vi "helper-collect-wind-direction.vi"(8 "error in":errorcluster, 10 "Result Virtual Name":string, 11 "Value in":dbl) -> (0 "error out":errorcluster, 1 "BUF Node":T1={"ADDR"=0, "Label"="", "Type"=enum."DI", "Mode"=enum."RIO", "Value"="", "Tags"="", "calibration"=[]} {"calibration"."Y" format="%#.3f"; "calibration"."X" format="%#.3f"; "ADDR" format="%04d"}, 2 "Result Node":T1={"ADDR"=0, "Label"="", "Type"=enum."DI", "Mode"=enum."RIO", "Value"="", "Tags"="", "calibration"=[]} {"calibration"."Y" format="%#.3f"; "calibration"."X" format="%#.3f"; "ADDR" format="%04d"}, 3 "Result":dbl)   [LabVIEW 2024]
uses:
  controls/IONode.ctl
  controls/type.address.ctl
  controls/enum.io.type.ctl
  controls/enum.io.mode.ctl
  controls/typeXyPoint.ctl
  controls/enumVarCtrlIO.ctl
  <vilib>/Utility/error.llb/Trim Whitespace.vi
  <vilib>/Utility/error.llb/Trim Whitespace One-Sided.vi
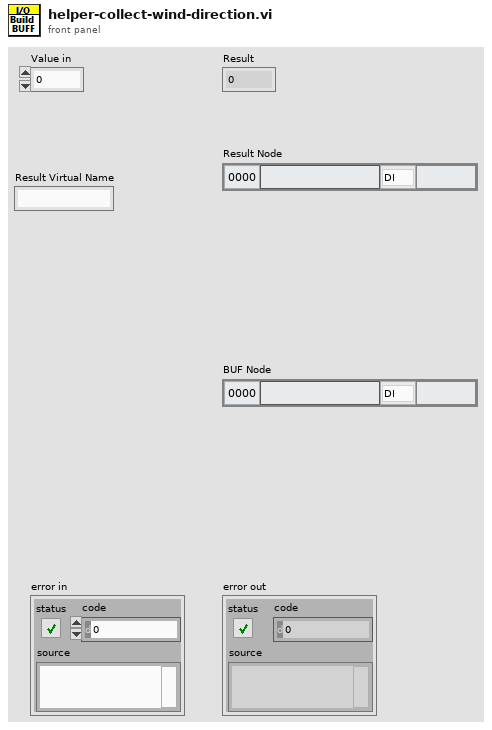
[diagram p1: front panel]
types:
  T1 = typedef "IONode.ctl" = cluster{"ADDR":T2, "Label":string, "Type":T3, "Mode":T4, "Value":string, "Tags":string, "calibration":T5[]}
  T2 = typedef "type.address.ctl" = u16
  T3 = typedef "enum.io.type.ctl" = enum16{"Type", "DI", "DO", "AI", "AO", "VL", "BUF"}
  T4 = typedef "enum.io.mode.ctl" = enum16{"Mode", "RIO", "SIM"}
  T5 = typedef "typeXyPoint.ctl" = cluster{"X":dbl, "Y":dbl}
  T6 = typedef "enumVarCtrlIO.ctl" = enum16{"IO Get By Key", "IO List Configs", "IO Add By Key", "IO Modify Value By Key", "IO Modify Calib By Key", "IO Modify ADDR By Key", "IO Modify Mode By Key", "IO Modify Type By Key", "IO Modify Name By Key", "IO Remove By Key", "IO Remove All"}
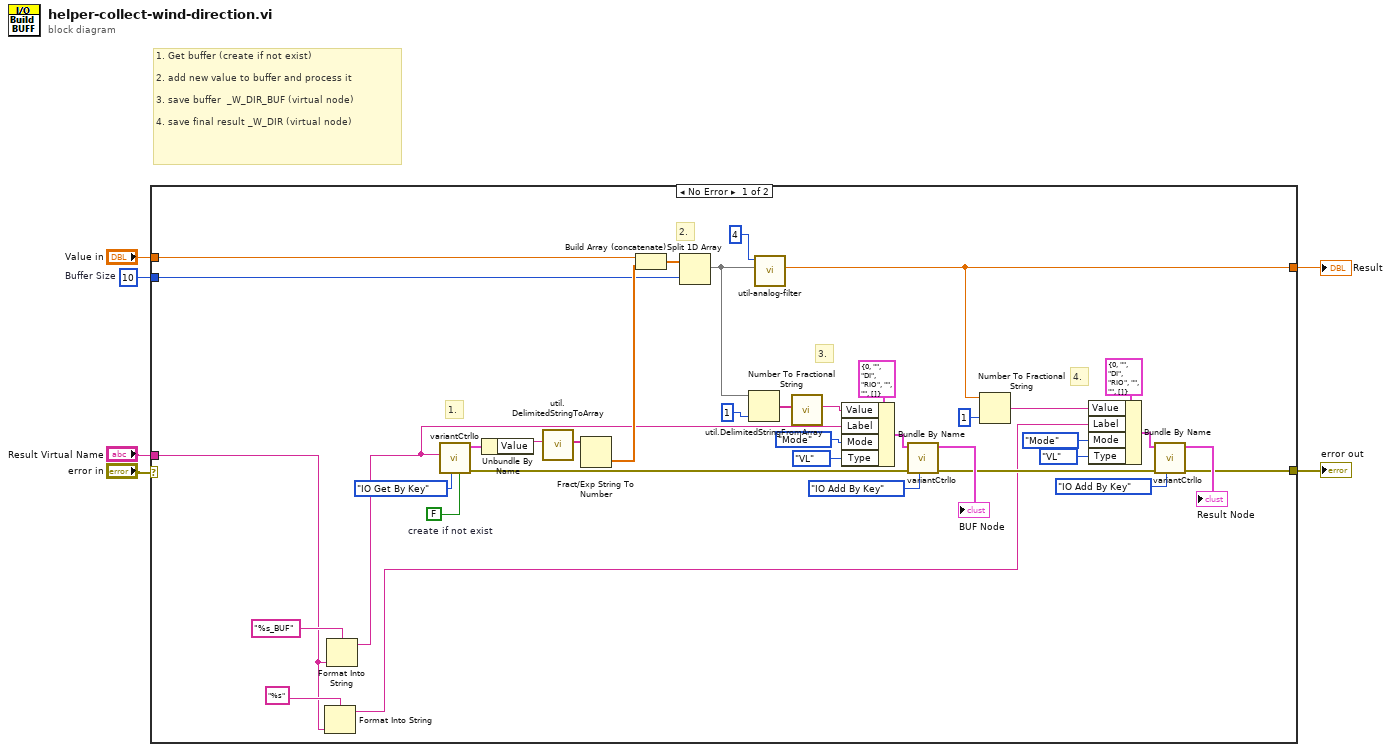
[diagram p0: block diagram]
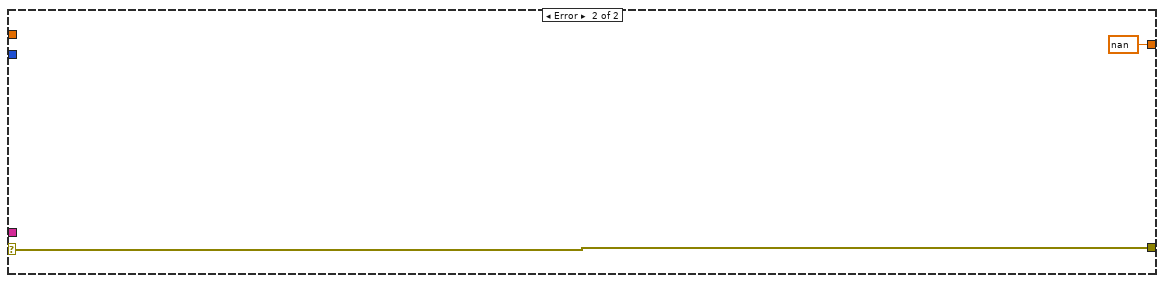
[diagram p2: hidden frame]
diagram:
  w1 = 10  # Buffer Size
  # "1. Get buffer (create if not exist)\n\n2. add new value to buffer and process it \n\n3. save buffer  _W_DIR_BUF (virtual node)\n\n4. save final result _W_DIR (virtual node)"
  n1 = case shown="No Error" "error in" {
    selector: "error in" -> [_ w45]
    tunnel: [w20 w45] -> w6
    tunnel: [w15 nan ("Filtered Value")] -> w4
    tunnel: "Result Virtual Name" -> [w7 _]
    tunnel: "Value in" -> [w13 _]
    tunnel: w1 -> [w12 _]
    frame No Error {
      w41 = FALSE  # create if not exist
      # "4."
      # "3."
      # "2."
      # "1."
      n2 = Format Into String(format string="%s", w7) -> (resulting string=w8:string)  [unwired: 2 in, 1 out]
      n3 = Format Into String(format string="%s_BUF", w7) -> (resulting string=w9:string)  [unwired: 2 in, 1 out]
      n4 = call "variantCtrlIo.vi"("isRequired (T)"=w41, "menu (Get Param)"=enumVarCtrlIO."IO Get By Key", "Key (use IOnode Label if empty )"=w9) -> ("error out"=w38:errorcluster, "IOnode out"=w43:T1)  [unwired: 4 in, 3 out]
      n5 = Unbundle By Name(w43) -> ("Value"=w42:string)
      n6 = call "util.DelimitedStringToArray.vi"("delimitaed string"=w42) -> ("array out"=w19:string[])  [unwired: 10 in]
      n7 = Fract/Exp String To Number(string=w19) -> (number=w18:dbl[])  [unwired: 3 in, 1 out]
      n8 = Build Array (concatenate)(w13, w18) -> (w40:dbl[])
      n9 = Split 1D Array(array=w40, index=w12) -> (first subarray=w17:dbl[])  [unwired: 1 out]
      n10 = Number To Fractional String(number=w17, precision (6)=i16 1) -> (F-format string=w16:string[])  [unwired: 2 in]
      n11 = call "util-analog-filter.vi"("Array"=w17, "# of mins&maxs to remove"=4) -> ("Filtered Value"=w15:dbl)  [unwired: 9 in]
      n12 = call "util.DelimitedStringFromArray.vi"("params array in"=w16) -> ("delimited string out"=w35:string)  [unwired: 10 in]
      n13 = Bundle By Name(cluster=T1 {"ADDR"=0, "Label"="", "Type"=enum."DI", "Mode"=enum."RIO", "Value"="", "Tags"="", "calibration"=[]} ("IoConf in"), "Value"=w35, "Label"=w9, "Mode"=enum.io.mode."Mode", "Type"=enum.io.type."VL" ("type")) -> (w34:T1)
      n14 = call "variantCtrlIo.vi"("menu (Get Param)"=enumVarCtrlIO."IO Add By Key" ("menu in (get)"), "error in"=w38, "IOnode in"=w34) -> ("error out"=w21:errorcluster, "IOnode out"=→"BUF Node":T1)  [unwired: 4 in, 3 out]
      n15 = Number To Fractional String(number=w15, precision (6)=i16 1) -> (F-format string=w22:string)  [unwired: 2 in]
      n16 = Bundle By Name(cluster=T1 {"ADDR"=0, "Label"="", "Type"=enum."DI", "Mode"=enum."RIO", "Value"="", "Tags"="", "calibration"=[]} ("IoConf in"), "Value"=w22, "Label"=w8, "Mode"=enum.io.mode."Mode", "Type"=enum.io.type."VL" ("type")) -> (w26:T1)
      n17 = call "variantCtrlIo.vi"("menu (Get Param)"=enumVarCtrlIO."IO Add By Key" ("menu in (get)"), "error in"=w21, "IOnode in"=w26) -> ("error out"=w20:errorcluster, "IOnode out"=→"Result Node":T1)  [unwired: 4 in, 3 out]
    }
    frame Error {
    }
  }
  "error out" <- w6
  "Result" <- w4
